vi "Get Scatter Data.vi"(8 "error in":errorcluster, 11 "Neph in":refnum<class "Nephelometer.lvclass">) -> (0 "error out":errorcluster, 2 "Data Record":T1, 3 "Neph out":refnum<class "Nephelometer.lvclass">)   [LabVIEW 2014, in "Nephelometer.lvclass"]
uses:
  Nephelometer.lvclass
  Nephelometer.lvclass/Nephelometer.ctl
  Reusable/Session APIs/Serial/Public/Get Data/Get String.vi
  Reusable/Session APIs/Text Communication/Text Device Session.lvclass
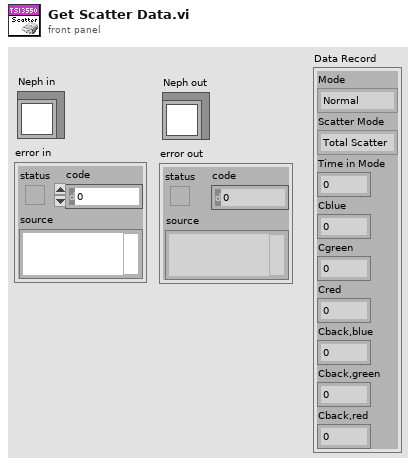
[diagram p1: front panel]
types:
  T1 = cluster{"Mode":enum16{"Normal", "Zero", "Blank"}, "Scatter Mode":enum16{"Total Scatter", "Back Scatter"}, "Time in Mode":i32, "Cblue":dbl, "Cgreen":dbl, "Cred":dbl, "Cback,blue":dbl, "Cback,green":dbl, "Cback,red":dbl}
  T2 = typedef "Session - Root.lvclass/Session Handle.ctl" = refnum<data-value>
  T3 = cluster{enum16{"Normal", "Zero", "Blank"}, enum16{"Total Scatter", "Back Scatter"}, i32, dbl, dbl, dbl, dbl, dbl, dbl}
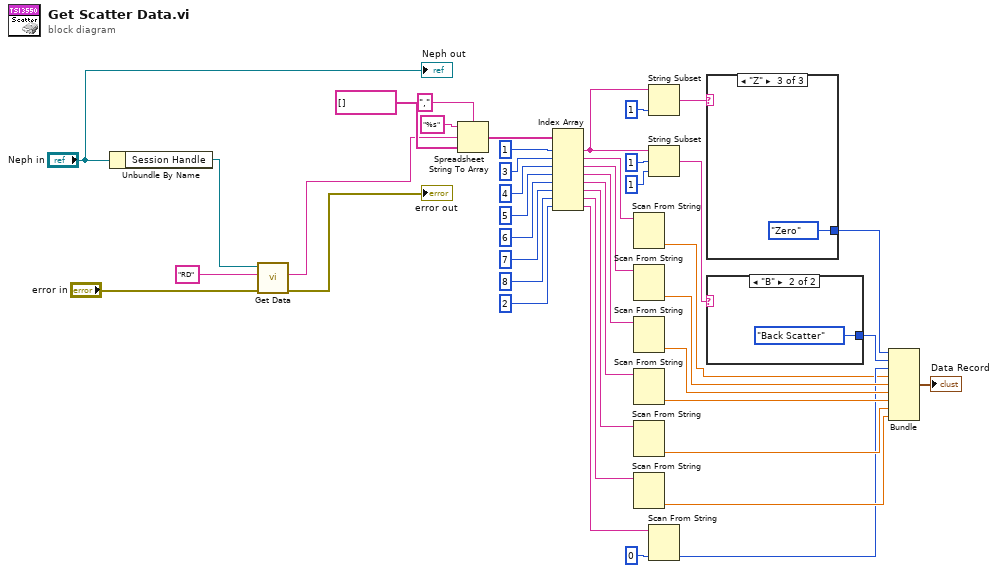
[diagram p0: block diagram]
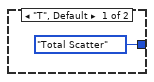
[diagram p2: hidden frame]
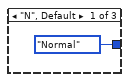
[diagram p3: hidden frame]
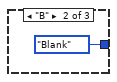
[diagram p4: hidden frame]
diagram:
  n1 = Unbundle By Name("Neph in") -> ("Session Handle"=w4:T2)
  n2 = call-poly "Get Data.vi"("error in"="error in", "CMD"="RD", "handle in"=w4) -> ("error out"=→"error out":errorcluster, "DataOut"=w1:string)  [unwired: 6 in, 1 out]
  n3 = Spreadsheet String To Array(delimiter (Tab)=",", format string="%s", spreadsheet string=w1, array type (2D Dbl)=string[] []) -> (array=w38:string[])
  n4 = Index Array(array=w38, index #1=1 ("index"), index #2=3 ("index"), index #3=4 ("index"), index #4=5 ("index"), index #5=6 ("index"), index #6=7 ("index"), index #7=8 ("index"), index #8=2 ("index")) -> (element #1=w32:string, element #2=w27:string, element #3=w25:string, element #4=w22:string, element #5=w18:string, element #6=w16:string, element #7=w13:string, element #8=w10:string)
  n5 = Scan From String(input string=w27) -> (output 1=w6:dbl)  [unwired: 4 in, 3 out]
  n6 = Scan From String(input string=w25) -> (output 1=w24:dbl)  [unwired: 4 in, 3 out]
  n7 = Scan From String(input string=w22) -> (output 1=w21:dbl)  [unwired: 4 in, 3 out]
  n8 = Scan From String(input string=w18) -> (output 1=w17:dbl)  [unwired: 4 in, 3 out]
  n9 = Scan From String(input string=w16) -> (output 1=w15:dbl)  [unwired: 4 in, 3 out]
  n10 = Scan From String(input string=w13) -> (output 1=w12:dbl)  [unwired: 4 in, 3 out]
  n11 = String Subset(string=w32, length (rest)=1 ("length (rest)")) -> (substring=w33:string)  [unwired: 1 in]
  n12 = String Subset(string=w32, offset (0)=1, length (rest)=1 ("length (rest)")) -> (substring=w29:string)
  n13 = Scan From String(input string=w10, default 1=0) -> (output 1=w7:i32)  [unwired: 3 in, 3 out]
  n14 = case shown="\"Z\"" w33 {
    tunnel: [enum16{"Normal", "Zero", "Blank"}."Normal" enum16{"Normal", "Zero", "Blank"}."Blank" enum16{"Normal", "Zero", "Blank"}."Zero"] -> w36
    frame "N", Default {
    }
    frame "B" {
    }
    frame "Z" {
    }
  }
  n15 = case shown="\"B\"" w29 {
    tunnel: [enum16{"Total Scatter", "Back Scatter"}."Total Scatter" enum16{"Total Scatter", "Back Scatter"}."Back Scatter"] -> w35
    frame "T", Default {
    }
    frame "B" {
    }
  }
  n16 = Bundle(w36, w35, w7, w6, w24, w21, w17, w15, w12) -> (→"Data Record":T3)  [unwired: 1 in]
  "Neph out" <- "Neph in"
